vi "CBL Node Check.vi"(7 "TimeOut":u32, 8 "error in (no error)":errorcluster, 9 "NodeAddr":u8, 10 "CANIndex":i32, 11 "DevIndex":i32) -> (0 "error out":errorcluster, 1 "function return":i32, 2 "pType":u32, 3 "pVersion":u32)   [LabVIEW 2012, in "CANBootloader.lvlib"]
doc: "int WINAPI CBL_NodeCheck(int DevIndex,int CANIndex,unsigned char NodeAddr,unsigned int *pVersion,unsigned int *pType,unsigned int TimeOut);"
uses:
  CANBootloader.lvlib
  Ginkgo_Driver.dll
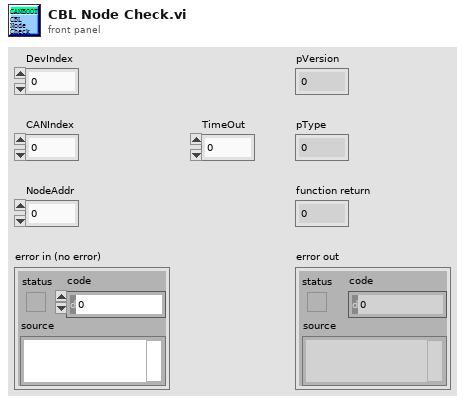
[diagram p1: front panel]
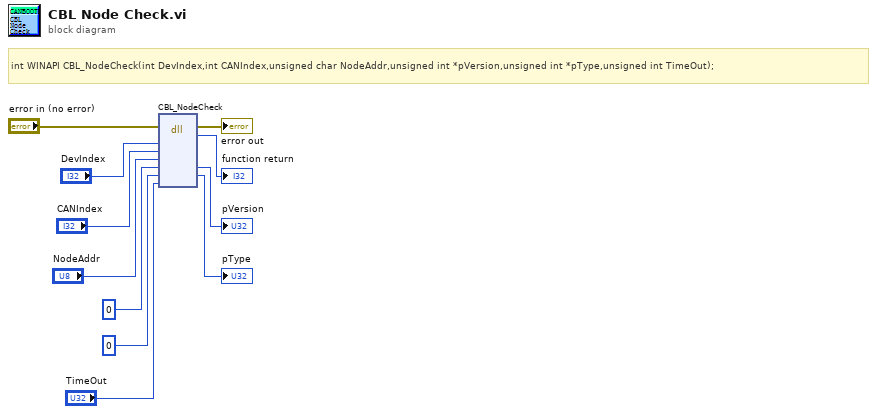
[diagram p0: block diagram]
diagram:
  # "int WINAPI CBL_NodeCheck(int DevIndex,int CANIndex,unsigned char NodeAddr,unsigned int *pVersion,unsigned int *pType,unsigned int TimeOut);"
  n1 = dll-call lib="E:/Project/vt_ginkgo/truck/Ginkgo Driver/vs2010/Ginkgo_USB-I2C_API_v2.0.3.0/lib/labview_64bit/CANBootloader/Ginkgo_Driver.*" fn="CBL_NodeCheck"(error in="error in (no error)", "DevIndex"="DevIndex", "CANIndex"="CANIndex", "NodeAddr"="NodeAddr", "pVersion"=u32 0, "pType"=u32 0, "TimeOut"="TimeOut") -> (error out=→"error out":errorcluster, →"function return":i32, "pVersion"=→"pVersion":u32, "pType"=→"pType":u32)  [unwired: 6 in, 1 out]
